vi "Asynchronous Call and Collect.vi"() -> ()   [LabVIEW 2014]
doc: "This VI demonstrates an asynchronous call and collecting the outputs later.\n\nWhen this VI is run, it asynchronously calls a target VI and will wait for the results in a different location. \n\nThis example uses the Start Asynchronous Call method and the Open VI Reference option 0x100."
panel:
  out "current time":timestamp
  in  "Collect":bool
  out "X + Y":dbl
  in  "Y":dbl=2.0
  in  "X":dbl=1.0
  # "Overview: Demonstrates the use of the call and collect option (0x100) with Asynchronous VI Calls.\nInstructions:\nRun the VI. Observe the behavior of the VI being called asynchronously. See the block diagram for more information."
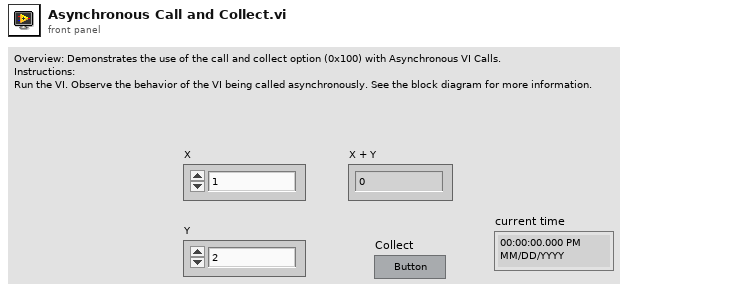
[diagram p1: front panel]
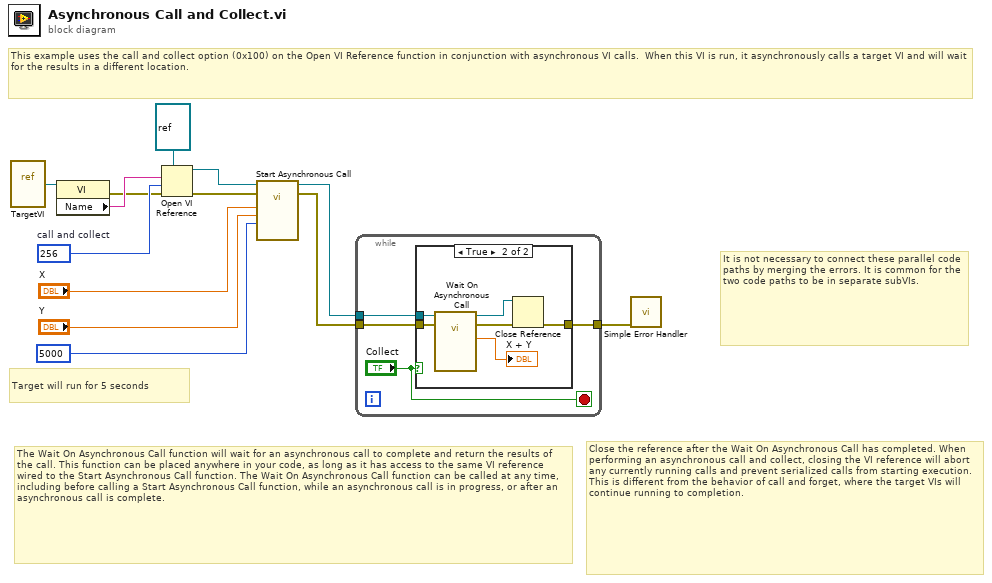
[diagram p0: block diagram]
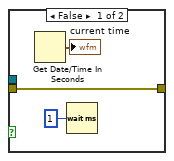
[diagram p2: hidden frame]
diagram:
  w13 = 256  # call and collect
  # "This example uses the call and collect option (0x100) on the Open VI Reference function in conjunction with asynchronous VI calls.  When this VI is run, it asynchronously calls a target VI and will wait for the results in a different location."
  # "It is not necessary to connect these parallel code paths by merging the errors. It is common for the two code paths to be in separate subVIs."
  # "Close the reference after the Wait On Asynchronous Call has completed. When performing an asynchronous call and collect, closing the VI reference will abort any currently running calls and prevent serialized calls from starting execution. This is different from the behavior of call and forget, where the target VIs will continue running to completion."
  # "The Wait On Asynchronous Call function will wait for an asynchronous call to complete and return the results of the call. This function can be placed anywhere in your code, as long as it has access to the same VI reference wired to the Start Asynchronous Call function. The Wait On Asynchronous Call function can be called at any time, including before calling a Start Asynchronous Call function, while an asynchronous call is in progress, or after an asynchronous call is complete."
  # "Target will run for 5 seconds"
  n1 = vi-ref "TargetVI.vi"() -> (w11:refnum<vi>)
  n2 = property class="VI"(reference=w11) -> (error out=w5:errorcluster, "Name"=w10:string)  [unwired: 1 in, 1 out]
  n3 = Open VI Reference(type specifier VI Refnum (for type only)=refnum<vi> refnum, vi path=w10, options=w13, error in (no error)=w5) -> (vi reference=w8:refnum<vi>, error out=w9:errorcluster)  [unwired: 2 in]
  n4 = call-by-ref "Start Asynchronous Call"(reference=w8, error in=w9, "Wait (ms)"=u32 5000 ("Wait (Milliseconds)"), "Y"="Y", "X"="X") -> (reference out=w3:refnum<vi>, error out=w2:errorcluster)  [unwired: 8 in, 1 out]
  n5 = while {
    tunnel: w3 -> [w17]
    tunnel: w2 -> [w16]
    tunnel: [w14] -> w1
    stop <- "Collect" stop-if-true
    n6 = case shown="True" "Collect" {
      tunnel: w17 -> [_ w23]
      tunnel: w16 -> [w18 w22]
      tunnel: [w18 w21] -> w14
      frame False {
        n7 = Get Date/Time In Seconds() -> (seconds since 1Jan1904=→"current time":timestamp)
        n8 = Wait (ms)(milliseconds to wait=u32 1) -> ()  [unwired: 1 out]
      }
      frame True {
        n9 = call-by-ref "Wait On Asynchronous Call"(reference=w23, error in=w22) -> (reference out=w26:refnum<vi>, error out=w25:errorcluster, "X + Y"=→"X + Y":dbl)  [unwired: 11 in]
        n10 = Close Reference(reference=w26, error in (no error)=w25) -> (error out=w21:errorcluster)
      }
    }
  }
  n11 = call <vilib>:"Simple Error Handler.vi"("error in (no error)"=w1) -> ()  [unwired: 4 in, 5 out]
